vi "oa_Buffer Update Value.vi"(4 "buffer speed profile?":bool, 5 "current speed profile":cluster{"time [s]":dbl[], "speed [rpm]":dbl[]}, 6 "number of spectra (40)":i32=40 min=1, 7 "previeous speed profile":cluster{"time [s]":dbl[], "speed [rpm]":dbl[]}, 8 "current offset":dbl=5250.0, 9 "current multiplier":dbl=50.0, 10 "current value":dbl[][](array[numeric])=array16x1024[16384 elements], 11 "previous value":dbl[][](array[numeric])=array85x1024[87040 elements]) -> (1 "speed profile":cluster{"time [s]":dbl[], "speed [rpm]":dbl[]}, 2 "Offset":dbl=1050.0, 3 "value":dbl[][](array[numeric]))   [LabVIEW 2017]
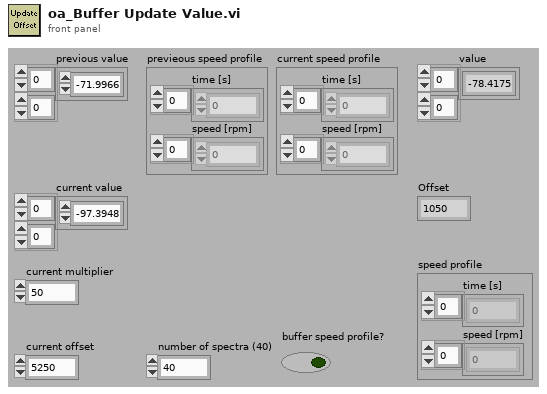
[diagram p1: front panel]
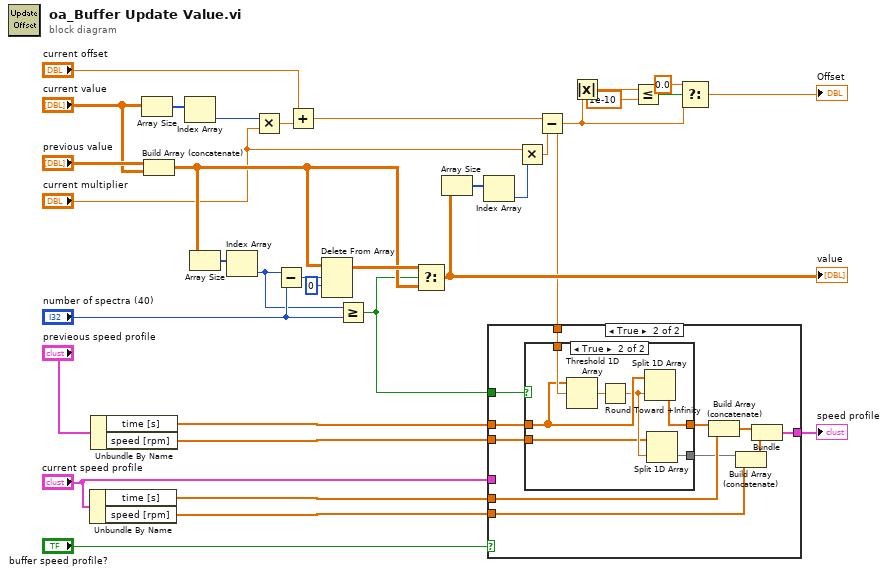
[diagram p0: block diagram]
diagram:
  n1 = Unbundle By Name("current speed profile") -> ("time [s]"=w10:dbl[], "speed [rpm]"=w9:dbl[])
  n2 = Unbundle By Name("previeous speed profile") -> ("time [s]"=w13:dbl[], "speed [rpm]"=w11:dbl[])
  n3 = Array Size(array="current value") -> (size(s)=w24:i32[])
  n4 = Build Array (concatenate)("previous value", "current value") -> (w31:dbl[][])
  n5 = Index Array(array=w24) -> (element=w23:i32)  [unwired: 1 in]
  n6 = Array Size(array=w31) -> (size(s)=w34:i32[])
  n7 = Index Array(array=w34) -> (element=w17:i32)  [unwired: 1 in]
  n8 = Multiply(x=w23, y="current multiplier") -> (x*y=w21:dbl)
  n9 = Subtract(x=w17, y="number of spectra (40)") -> (x-y=w14:i32)
  n10 = Add(x="current offset", y=w21) -> (x+y=w22:dbl)
  n11 = Delete From Array(array=w31, length=w14, index (row)=0) -> (array with subset deleted=w33:dbl[][])  [unwired: 1 in, 1 out]
  n12 = Greater Or Equal?(x=w17, y="number of spectra (40)") -> (x >= y?=w12:bool)
  n13 = Select(t=w33, s=w12, f=w31) -> (s? t:f=w29:dbl[][])
  "value" <- w29
  n14 = Array Size(array=w29) -> (size(s)=w28:i32[])
  n15 = Index Array(array=w28) -> (element=w27:i32)  [unwired: 1 in]
  n16 = Multiply(x="current multiplier", y=w27) -> (x*y=w26:dbl)
  n17 = Subtract(x=w22, y=w26) -> (x-y=w3:dbl)
  n18 = case shown="True" "buffer speed profile?" {
    tunnel: [w35 w46] -> w15
    tunnel: w3 -> [_ w45]
    tunnel: w13 -> [_ w44]
    tunnel: w12 -> [_ w43]
    tunnel: w11 -> [_ w42]
    tunnel: w10 -> [_ w40]
    tunnel: w9 -> [_ w38]
    tunnel: "current speed profile" -> [w35 _]
    frame False {
    }
    frame True {
      n19 = case shown="True" w43 {
        tunnel: w45 -> [_ w55]
        tunnel: w44 -> [w48 w53]
        tunnel: w42 -> [w47 w51]
        tunnel: [w48 w50] -> w41
        tunnel: [w47 w49] -> w39
        frame False {
        }
        frame True {
          n20 = Threshold 1D Array(2:w55, 3:w53) -> (0:w54:dbl)  [unwired: 1 in]
          n21 = Round Toward +Infinity(x=w54) -> (ceil(x): smallest int >= x=w52:dbl)
          n22 = Split 1D Array(array=w53, index=w52) -> (second subarray=w50:dbl[])  [unwired: 1 out]
          n23 = Split 1D Array(array=w51, index=w52) -> (second subarray=w49:dbl[])  [unwired: 1 out]
        }
      }
      n24 = Build Array (concatenate)(w41, w40) -> (w37:dbl[])
      n25 = Build Array (concatenate)(w39, w38) -> (w36:dbl[])
      n26 = Bundle(w37, w36) -> (w46:cluster{dbl[], dbl[]})  [unwired: 1 in]
    }
  }
  "speed profile" <- w15
  n27 = Absolute Value(x=w3) -> (abs(x)=w6:dbl)
  n28 = Less Or Equal?(x=w6, y=1e-10) -> (x <= y?=w5:bool)
  n29 = Select(t=0.0, s=w5, f=w3) -> (s? t:f=→"Offset":dbl)
